vi "IsDLLPathSDL.vi"(11 "DLL Path":path) -> (0 "Lib Folder":path, 1 "Platform Type":T1=enum."Win32", 2 "Library Name":string, 3 "Is SDL?":bool)   [LabVIEW 2024, in "CustomActions.lvlib"]
uses:
  CustomActions.lvlib
  PlatformType--enum.ctl
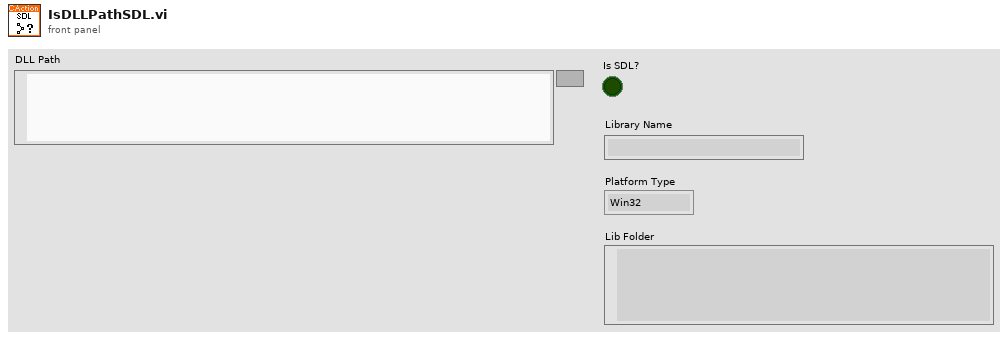
[diagram p1: front panel]
types:
  T1 = typedef "CustomActions.lvlib/PlatformType--enum.ctl" = enum16{"Unknown", "Win32", "Win64", "Linux64"}
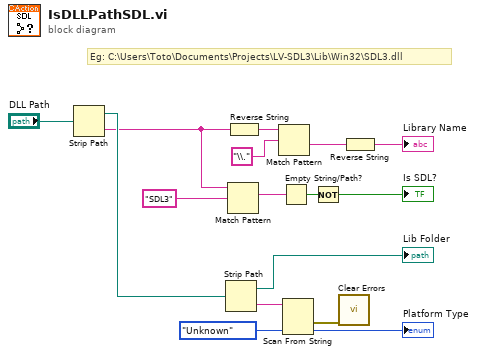
[diagram p0: block diagram]
diagram:
  # "Eg: C:\\Users\\Toto\\Documents\\Projects\\LV-SDL3\\Lib\\Win32\\SDL3.dll"
  n1 = Strip Path(path="DLL Path") -> (stripped path=w11:path, name=w7:string)
  n2 = Strip Path(path=w11) -> (stripped path=→"Lib Folder":path, name=w10:string)
  n3 = Match Pattern(string=w7, regular expression="SDL3") -> (match substring=w14:string)  [unwired: 1 in, 3 out]
  n4 = Reverse String(1:w7) -> (0:w5:string)
  n5 = Match Pattern(string=w5, regular expression="\\.") -> (after substring=w3:string)  [unwired: 1 in, 3 out]
  n6 = Empty String/Path?(string/path=w14) -> (empty?=w13:bool)
  n7 = Scan From String(input string=w10, default 1=PlatformType--enum."Unknown" ("Lib Type")) -> (error out=w6:errorcluster, output 1=→"Platform Type":T1)  [unwired: 3 in, 2 out]
  n8 = Not(x=w13) -> (.not. x?=→"Is SDL?":bool)
  n9 = call <vilib>:"Clear Errors.vi"("error in (no error)"=w6) -> ()  [unwired: 5 in, 2 out]
  n10 = Reverse String(1:w3) -> (0:→"Library Name":string)
